vi "ColorSpecification.vi"(10 "Color":T1) -> (3 "ColorSpecification":refnum<class "ColorSpecification.lvclass">)   [LabVIEW 2018, in "ColorSpecification.lvclass"]
uses:
  ColorSpecification.lvclass
  Product/Color.ctl
  ColorSpecification.lvclass/ColorSpecification.ctl
  Product/Product.lvclass
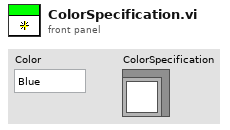
[diagram p1: front panel]
types:
  T1 = typedef "Product.lvclass/Color.ctl" = enum16{"Blue", "Green", "Red"}
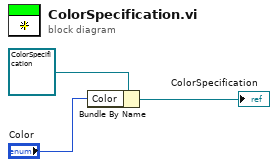
[diagram p0: block diagram]
diagram:
  n1 = Bundle By Name(cluster=refnum<class "ColorSpecification.lvclass"> refnum ("ColorSpecification.lvclass"), "Color"="Color") -> (→"ColorSpecification":refnum<class "ColorSpecification.lvclass">)
